vi "Append New Mappings.vi"(9 "Type":T1, 10 "Mappings to Append":T2(array[cluster]), 11 "Mappings in":T3[](array[typedef])) -> (3 "Mappings out":T3[](array[typedef]))   [LabVIEW 2013, in "Engine Runtime Interface.lvclass"]
uses:
  Engine Runtime Interface.lvclass
  Engine Configuration/Mappings.ctl
  <vilib>/NI/Tag Bus/tag/Data Type.ctl
  <vilib>/NI/Tag Bus/tag/tag descriptor.lvclass
  Engine Configuration/engine configuration.lvclass
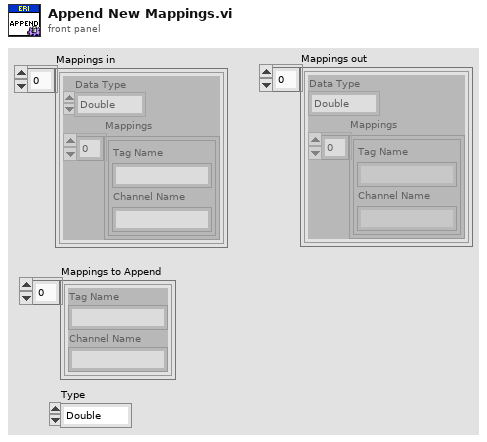
[diagram p1: front panel]
types:
  T1 = typedef "tag bus.lvlib/tag descriptor.lvclass/Data Type.ctl" = enum16{"Double", "Single", "I64", "I32", "I16", "I8", "U64", "U32", "U16", "U8", "Boolean", "String", "Array of Double", "Array of Single", "Array of I64", "Array of I32", "Array of I16", "Array of I8", "Array of U64", "Array of U32", "Array of U16", "Array of U8", "Array of Boolean", "Array of String"}
  T2 = cluster{"Tag Name":string, "Channel Name":string}[]
  T3 = typedef "engine configuration.lvclass/Mappings.ctl" = cluster{"Data Type":T1, "Mappings":cluster{"Tag Name":string, "Channel Name":string}[]}
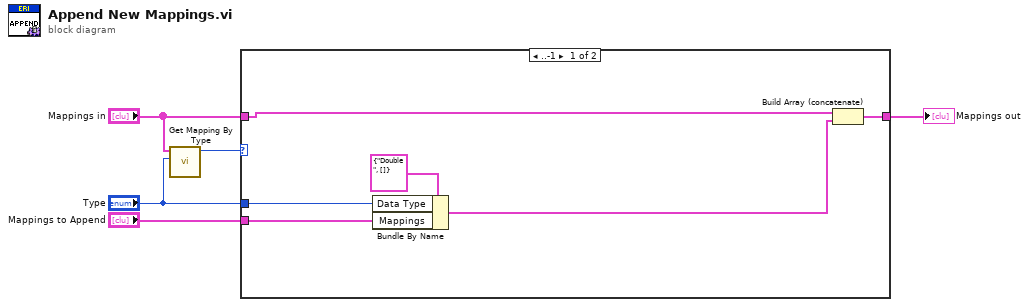
[diagram p0: block diagram]
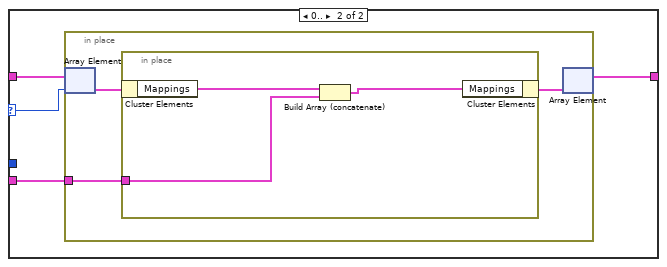
[diagram p2: hidden frame]
diagram:
  n1 = call "Get Mapping By Type.vi"("Type"="Type", "Mappings"="Mappings in") -> ("index"=w5:i32)  [unwired: 9 in]
  n2 = case shown="..-1" w5 {
    selector: w5 -> [_ w15]
    tunnel: "Mappings in" -> [w10 w14]
    tunnel: "Type" -> [w7 _]
    tunnel: "Mappings to Append" -> [w6 w12]
    tunnel: [w9 w13] -> w1
    frame ..-1 {
      n3 = Bundle By Name(cluster=T3 {"Data Type"=enum."Double", "Mappings"=[]} ("Mapping"), "Data Type"=w7, "Mappings"=w6) -> (w8:T3)
      n4 = Build Array (concatenate)(w10, w8) -> (w9:T3[])
    }
    frame 0.. {
      n5 = in-place {
        in-place-border: w12 -> [w16]
        n6 = in-place-array #1(w14, w15) -> (w18:T3)
        n7 = in-place {
          in-place-border: w16 -> [w20]
          n8 = in-place-cluster #2(w18) -> ("Mappings"=w21:T2)
          n9 = Build Array (concatenate)(w21, w20) -> (w19:T2)
          n10 = in-place-cluster #2("Mappings"=w19) -> (w17:T3)
        }
        n11 = in-place-array #1(w17) -> (w13:T3[])  [unwired: 1 out]
      }
    }
  }
  "Mappings out" <- w1
